vi "Go.vi"(9 "Timing Values":dbl[](array[numeric]), 10 "Control In":T1, 11 "CAD Dispense in":refnum<class "CAD Dispense.lvclass">) -> (2 "Control Out":T1, 3 "CAD Dispense Out":refnum<class "CAD Dispense.lvclass">)   [LabVIEW 2020, in "CAD Dispense.lvclass"]
uses:
  CAD Dispense.lvclass
  Controller/Controllers.ctl
  Controller/I-O/I-O.lvclass
  Controller/Dispenser/Dispenser.lvclass
  C:/Program Files (x86)/Aerotech/A3200/LabVIEW/2010/Bin/Aerotech.A3200.dll
  Program Files (x86)/Aerotech/A3200/LabVIEW/2010/Bin/Aerotech.A3200.dll
  CAD Dispense.lvclass/CAD Dispense.ctl
  Controller/Motion/Motion.lvclass
  Controller/Motion/A3200/A3200.lvclass
  Controller/Controller.lvclass
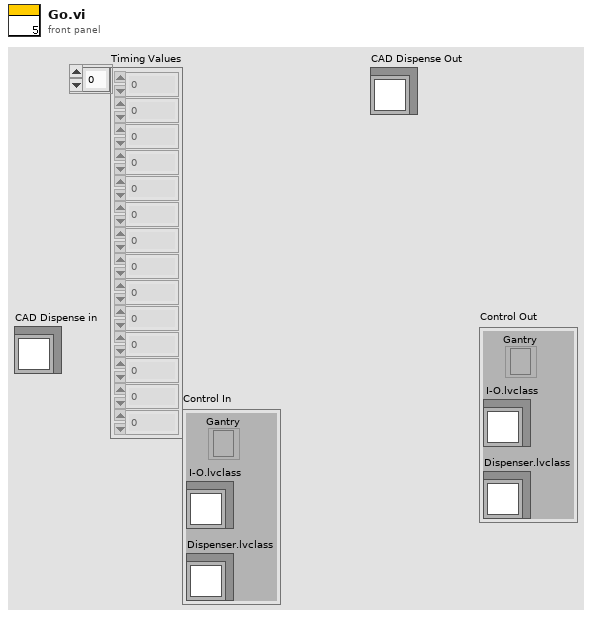
[diagram p1: front panel]
types:
  T1 = typedef "Controller.lvclass/Controllers.ctl" = cluster{"I-O.lvclass":refnum<class "I-O.lvclass">, "Dispenser.lvclass":refnum<class "Dispenser.lvclass">, "Gantry":refnum<k24>}
  T2 = cluster{"Motion":dbl[][], "Center":dbl[], "Circle?":bool, "CW/CCW":dbl}[]
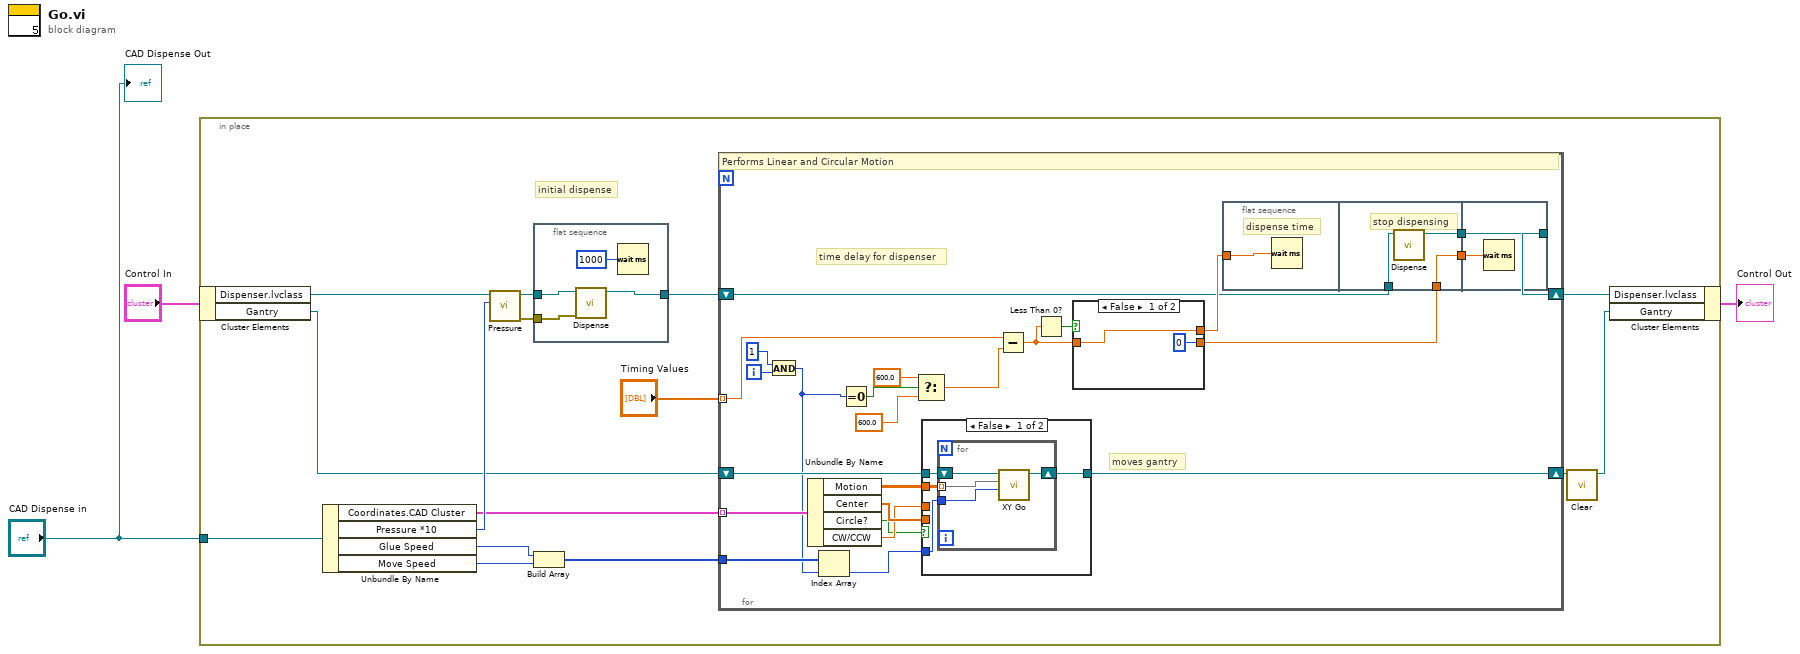
[diagram p0: block diagram]
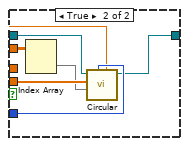
[diagram p2: hidden frame]
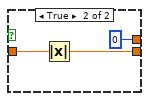
[diagram p3: hidden frame]
diagram:
  n1 = in-place {
    in-place-border: "CAD Dispense in" -> [w17]
    # "initial dispense"
    n2 = in-place-cluster #1("Control In") -> ("Dispenser.lvclass"=w11:refnum<class "Dispenser.lvclass">, "Gantry"=w5:refnum<k24>)
    n3 = Unbundle By Name(w17) -> ("Coordinates.CAD Cluster"=w7:T2, "Pressure *10"=w10:i64, "Glue Speed"=w15:i32, "Move Speed"=w14:i32)
    n4 = call-dynamic "Pressure.vi"("Pressure"=w10, "Dispenser in"=w11) -> ("error out"=w9:errorcluster, "Dispenser out"=w8:refnum<class "Dispenser.lvclass">)  [unwired: 8 in]
    n5 = flat-sequence {
      tunnel: [w20] -> w16
      tunnel: w9 -> [w19]
      tunnel: w8 -> [w21]
      frame #0 {
        n6 = call-dynamic "Dispense.vi"("error in (no error)"=w19, "Dispenser in"=w21) -> ("Dispenser out"=w20:refnum<class "Dispenser.lvclass">)  [unwired: 8 in, 1 out]
        n7 = Wait (ms)(milliseconds to wait=u32 1000) -> ()  [unwired: 1 out]
      }
    }
    n8 = Build Array(w15, w14) -> (w13:i32[])
    n9 = for {
      tunnel: w7 -> [w41] mode=indexing
      tunnel: "Timing Values" -> [w37] mode=indexing
      tunnel: w13 -> [w32]
      shift-right: [w34] -> w18
      shift-left: w16 -> [w42]
      shift-right: [w28] -> w6
      shift-left: w5 -> [w36]
      i -> [w31]
      # "time delay for dispenser"
      # "moves gantry"
      # "Performs Linear and Circular Motion"
      n10 = And(x=1, y=w31) -> (x .and. y?=w27:i32)
      n11 = Unbundle By Name(w41) -> ("Motion"=w40:dbl[][], "Center"=w39:dbl[], "Circle?"=w33:bool, "CW/CCW"=w35:dbl)
      n12 = Index Array(array=w32, index=w27) -> (element=w29:i32)
      n13 = Equal To 0?(x=w27) -> (x = 0?=w26:bool)
      n14 = Select(t=600.0, s=w26, f=600.0) -> (s? t:f=w23:dbl)
      n15 = case shown="False" w33 {
        tunnel: w35 -> [_ w57]
        tunnel: w40 -> [w51 w62]
        tunnel: w39 -> [_ w60]
        tunnel: w36 -> [w48 w61]
        tunnel: w29 -> [w50 w58]
        tunnel: [w49 w56] -> w28
        frame False {
          n16 = for {
            tunnel: w51 -> [w54] mode=indexing
            shift-right: [w52] -> w49
            shift-left: w48 -> [w55]
            tunnel: w50 -> [w53]
            n17 = call "XY Go.vi"("Speed"=w53, "XY"=w54, "Gantry 2"=w55) -> ("Gantry 3"=w52:refnum<k24>)  [unwired: 7 in, 1 out]
          }
        }
        frame True {
          n18 = Index Array(array=w62) -> (element=w59:dbl[])  [unwired: 2 in]
          n19 = call "Circular.vi"("Direction"=w57, "Speed"=w58, "XY End"=w59, "XY Center"=w60, "Gantry 2"=w61) -> ("Gantry 3"=w56:refnum<k24>)  [unwired: 5 in, 1 out]
        }
      }
      n20 = Subtract(x=w37, y=w23) -> (x-y=w38:dbl)
      n21 = Less Than 0?(x=w38) -> (x < 0?=w47:bool)
      n22 = case shown="False" w47 {
        tunnel: [w70 u32 0 ("milliseconds to wait")] -> w46
        tunnel: w38 -> [w70 w73]
        tunnel: [u32 0 ("milliseconds to wait") w72] -> w45
        frame False {
        }
        frame True {
          n23 = Absolute Value(x=w73) -> (abs(x)=w72:dbl)
        }
      }
      n24 = flat-sequence {
        tunnel: w46 -> [w63]
        tunnel: w42 -> [w65]
        tunnel: [w66] -> w44
        tunnel: w45 -> [w66]
        tunnel: [w64] -> w43
        tunnel: w44 -> [w68]
        tunnel: w43 -> [w67]
        tunnel: [w67] -> w34
        frame #0 {
          # "dispense time"
          n25 = Wait (ms)(milliseconds to wait=w63) -> ()  [unwired: 1 out]
        }
        frame #1 {
          # "stop dispensing"
          n26 = call-dynamic "Dispense.vi"("Dispenser in"=w65) -> ("Dispenser out"=w64:refnum<class "Dispenser.lvclass">)  [unwired: 9 in, 1 out]
        }
        frame #2 {
          n27 = Wait (ms)(milliseconds to wait=w68) -> ()  [unwired: 1 out]
        }
      }
    }
    n28 = call "Clear.vi"("Gantry 2"=w6) -> ("Gantry 3"=w4:refnum<k24>)  [unwired: 9 in, 1 out]
    n29 = in-place-cluster #1("Dispenser.lvclass"=w18, "Gantry"=w4) -> (→"Control Out":T1)
  }
  "CAD Dispense Out" <- "CAD Dispense in"
